vi "Close.vi"(8 "error in (no error)":errorcluster caption="entrée d'erreur (pas d'erreur)", 11 "Server TCP_IP (Default) en entrée":refnum<class "Server TCP_IP (Default).lvclass">) -> (0 "error out":errorcluster caption="sortie d'erreur", 3 "Server TCP_IP (Default) en sortie":refnum<class "Server TCP_IP (Default).lvclass">)   [LabVIEW 2020, in "Library Instrument & Equipement.lvlib" / "Library TCP IP.lvlib" / "Server TCP_IP (Default).lvclass"]
uses:
  Server TCP_IP (Default).lvclass
  Server TCP_IP (Default).lvclass/Server TCP_IP (Default).ctl
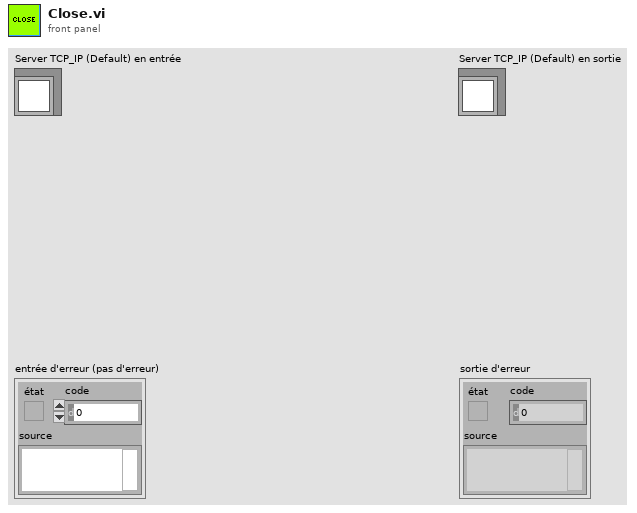
[diagram p1: front panel]
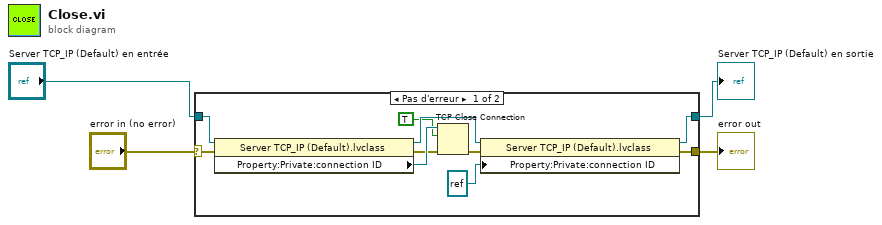
[diagram p0: block diagram]
diagram:
  n1 = case shown="Pas d'erreur" "error in (no error)" {
    selector: "error in (no error)" -> [w7 w16]
    tunnel: [w5 w16] -> w3
    tunnel: [w6 w15] -> w1
    tunnel: "Server TCP_IP (Default) en entrée" -> [w14 w15]
    frame No Error {
      n2 = property class="Server TCP_IP (Default).lvclass"(reference=w14, error in=w7) -> (reference out=w11:refnum<class "Server TCP_IP (Default).lvclass">, error out=w10:errorcluster, "Property:Private:connection ID"=w13:refnum<k5>)
      n3 = TCP Close Connection(connection ID=w13, abort (F)=TRUE ("abandonner (F)"), error in (no error)=w10) -> (error out=w9:errorcluster)  [unwired: 1 out]
      n4 = property class="Server TCP_IP (Default).lvclass"(reference=w11, error in=w9, "Property:Private:connection ID"=refnum<k5> refnum ("connection ID")) -> (reference out=w6:refnum<class "Server TCP_IP (Default).lvclass">, error out=w5:errorcluster)
    }
    frame Error {
    }
  }
  "error out" <- w3
  "Server TCP_IP (Default) en sortie" <- w1
